vi "Cross Spectrum (Mag-Phase).vi"(0 "time signal X":waveform(dbl), 1 "restart averaging (F)":bool, 2 "window parameter":dbl=nan, 5 "time signal Y":waveform(dbl), 7 "window":T1=1 items=["Rectangle"=0, "Hanning"=1, "Hamming"=2, "Blackman-Harris"=3, "Exact Blackman"=4, "Blackman"=5, "Flat Top"=6, "4 Term B-Harris "=7, "7 Term B-Harris"=8, "Low Sidelobe"=9, "Blackman Nuttall"=11, "Triangle"=30, "Bartlett-Hanning"=31, "Bohman"=32, "Parzen"=33, "Welch"=34, "Kaiser"=60, "Dolph-Chebyshev"=61, "Gaussian"=62], 9 "view":T3, 11 "error in (no error)":errorcluster, 12 "averaging parameters":T2={"averaging mode"=enum."No averaging", "weighting mode"=enum."Exponential", "number of averages"=10} {"number of averages" min=1}) -> (3 "averaging done":bool, 4 "magnitude":cluster{"f0":dbl, "df":dbl, "magnitude":dbl[]} {"magnitude" format="%.2p"; "f0" format="%0.2p"; "df" format="%0.2p"}, 6 "phase":cluster{"f0":dbl, "df":dbl, "phase":dbl[]} {"phase" format="%.2p"; "f0" format="%0.2p"; "df" format="%0.2p"}, 10 "averages completed":dbl format="%.2p", 15 "error out":errorcluster)   [LabVIEW 2020, in "NI_MAPro.lvlib"]
doc: "Computes the averaged cross power spectrum of the input signals. Results are returned as <B>magnitude</B> and <B>phase</B>."
uses:
  NI_MAPro.lvlib
  windowTd.ctl
  NI_AALPro.lvlib
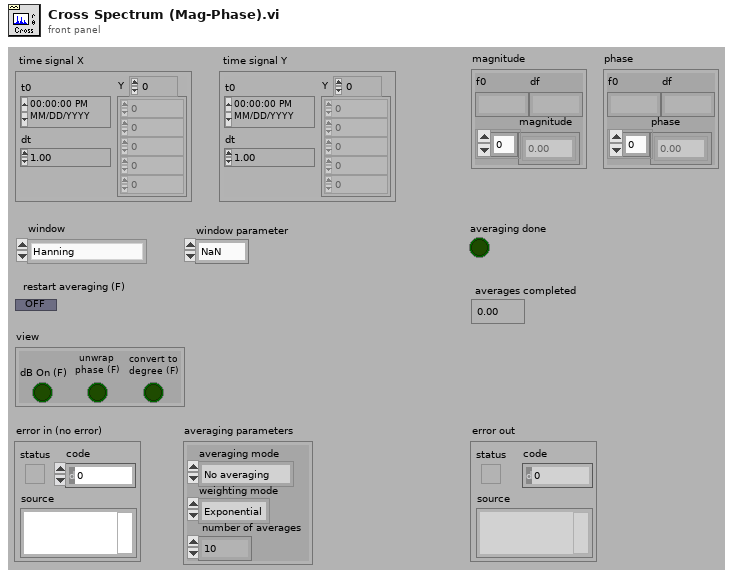
[diagram p1: front panel]
types:
  T1 = typedef "NI_AALPro.lvlib/windowTd.ctl" = u32
  T2 = cluster{"averaging mode":enum16{"No averaging", "Vector averaging", "RMS averaging", "Peak hold"}, "weighting mode":enum16{"Linear", "Exponential"}, "number of averages":u32}
  T3 = cluster{"dB On (F)":bool, "unwrap phase (F)":bool, "convert to degree (F)":bool}
  T4 = enum16{"FFT spectrum", "Power spectrum", "Cross spectrum", "Frequency response"}
  T5 = enum16{"No averaging", "Vector averaging", "RMS averaging", "Peak hold"}
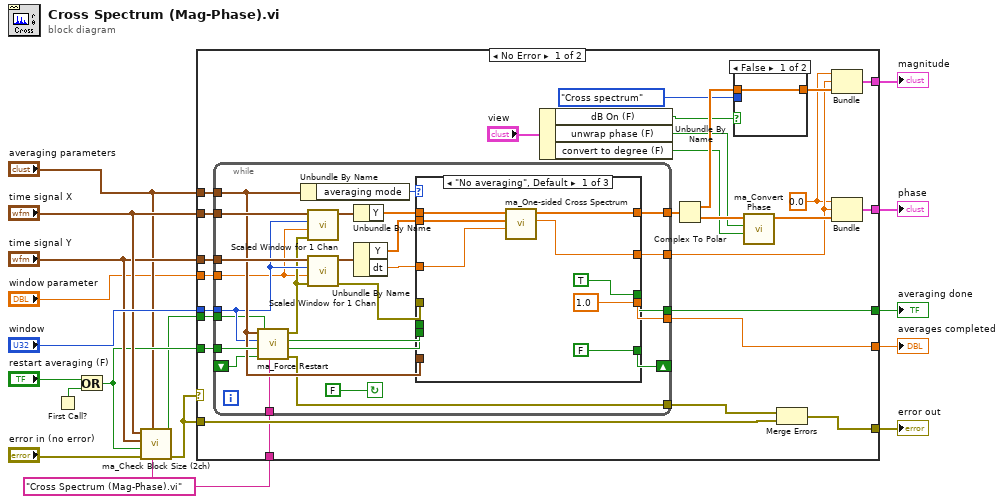
[diagram p0: block diagram]
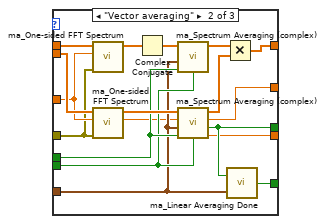
[diagram p2: hidden frame]
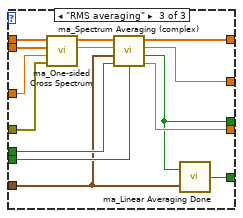
[diagram p3: hidden frame]
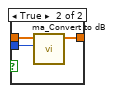
[diagram p4: hidden frame]
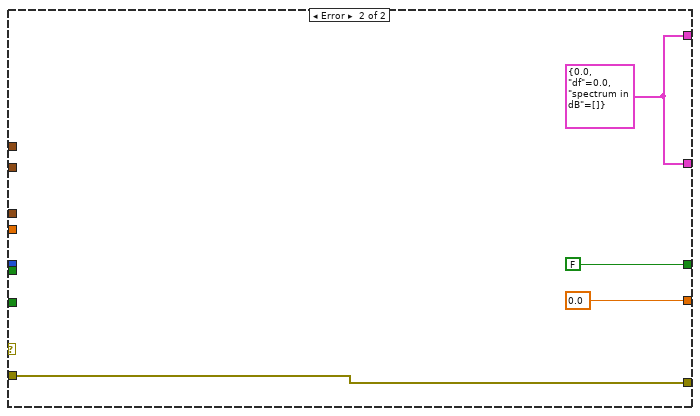
[diagram p5: hidden frame]
diagram:
  w3 = "Cross Spectrum (Mag-Phase).vi" ("caller VI name")
  n1 = First Call?() -> (First Call?: T/F=w7:bool)
  n2 = Or(x="restart averaging (F)", y=w7) -> (x .or. y?=w8:bool)
  n3 = call "ma_Check Block Size (2ch).vi"("caller VI name"=w3, "averaging parameters"="averaging parameters", "error in"="error in (no error)", "restart averaging (F)"=w8, "time signal Y"="time signal Y", "time signal X"="time signal X") -> ("error out"=w9:errorcluster, "force restart averaging"=w2:bool)  [unwired: 4 out]
  n4 = case shown="No Error" w9 {
    tunnel: "averaging parameters" -> [w43 _]
    tunnel: [w41 0.0 ("averages completed")] -> w17
    tunnel: "time signal X" -> [w40 _]
    tunnel: "time signal Y" -> [w39 _]
    tunnel: "window" -> [w38 _]
    tunnel: [w28 w115] -> w5
    tunnel: [w31 FALSE ("averaging done")] -> w15
    tunnel: w8 -> [w30 _]
    tunnel: [w23 w118] -> w14
    tunnel: w9 -> [w21 w118]
    tunnel: [w24 w115] -> w4
    tunnel: w3 -> [w20 _]
    tunnel: w2 -> [w19 _]
    tunnel: "window parameter" -> [w18 _]
    frame No Error {
      w25 = 0.0
      n5 = while {
        tunnel: w20 -> [w47]
        tunnel: [w48] -> w22
        tunnel: w30 -> [w62]
        shift-left: _ -> [w60]
        shift-right: [w64] -> _
        tunnel: [w65] -> w31
        tunnel: w38 -> [w52]
        tunnel: w39 -> [w66]
        tunnel: w40 -> [w67]
        tunnel: [w59] -> w26
        tunnel: [w68] -> w41
        tunnel: [w69] -> w42
        tunnel: w43 -> [w61]
        tunnel: w19 -> [w46]
        tunnel: w18 -> [w45]
        stop <- FALSE continue-if-true
        n6 = call "ma_Force Restart.vi"("caller VI name"=w47, "force restart averaging in"=w46, "linear averaging done"=w60, "restart averaging (F)"=w62, "window"=w52, "averaging parameters"=w61) -> ("error out"=w48:errorcluster, "retrieve last spectrum"=w49:bool, "force restart averaging"=w50:bool, "skip processing"=w51:errorcluster)  [unwired: 2 out]
        n7 = Unbundle By Name(w61) -> ("averaging mode"=w70:T5)
        n8 = call "Scaled Window for 1 Chan.vi"("error in (no error)"=w51, "window parameter"=w45, "window"=w52, "signal in"=w67) -> ("signal out"=w57:waveform(dbl))  [unwired: 5 in, 2 out]
        n9 = call "Scaled Window for 1 Chan.vi"("error in (no error)"=w51, "window parameter"=w45, "window"=w52, "signal in"=w66) -> ("error out"=w63:errorcluster, "signal out"=w53:waveform(dbl))  [unwired: 5 in, 1 out]
        n10 = Unbundle By Name(w57) -> ("Y"=w56:dbl[])
        n11 = Unbundle By Name(w53) -> ("Y"=w55:dbl[], "dt"=w54:dbl)
        n12 = case shown="\"No averaging\", Default" w70 {
          tunnel: w56 -> [w77 w95 w110]
          tunnel: w55 -> [w76 w93 w109]
          tunnel: w54 -> [w75 w92 w108]
          tunnel: [w73 w80 w97] -> w59
          tunnel: [w74 w96 w105] -> w69
          tunnel: w50 -> [_ w88 w106]
          tunnel: w61 -> [_ w83 w101]
          tunnel: [1.0 ("averages completed") w79 w99] -> w68
          tunnel: [TRUE ("averaging done") w82 w98] -> w65
          tunnel: [FALSE ("linear averaging done") w86 w104] -> w64
          tunnel: w63 -> [_ w85 w103]
          tunnel: w49 -> [_ w84 w102]
          frame "No averaging", Default {
            n13 = call "ma_One-sided Cross Spectrum.vi"("dt"=w75, "signal Y (V)"=w76, "signal X (V)"=w77) -> ("df"=w73:dbl, "cross spectrum (V^2 rms)"=w74:cdb[])  [unwired: 1 in, 6 out]
          }
          frame "Vector averaging" {
            n14 = call "ma_One-sided FFT Spectrum.vi"("error in"=w85, "dt"=w92, "signal (V)"=w95) -> ("FFT spectrum (Vrms)"=w94:cdb[])  [unwired: 8 out]
            n15 = call "ma_One-sided FFT Spectrum.vi"("error in"=w85, "dt"=w92, "signal (V)"=w93) -> ("df"=w81:dbl, "FFT spectrum (Vrms)"=w89:cdb[])  [unwired: 7 out]
            n16 = Complex Conjugate(1:w94) -> (0:w91:cdb[])
            n17 = call "ma_Spectrum Averaging (complex).vi"("complex spectrum"=w91, "retrieve last spectrum (F)"=w84, "averaging parameters"=w83, "restart averaging (F)"=w88) -> ("averaged complex spectrum"=w90:cdb[])  [unwired: 1 in, 4 out]
            n18 = call "ma_Spectrum Averaging (complex).vi"("complex spectrum"=w89, "df"=w81, "retrieve last spectrum (F)"=w84, "averaging parameters"=w83, "restart averaging (F)"=w88) -> ("averaged complex spectrum"=w87:cdb[], "df"=w80:dbl, "averaging done"=w82:bool, "averages completed"=w79:dbl)  [unwired: 1 out]
            n19 = Multiply(x=w90, y=w87) -> (x*y=w96:cdb[])
            n20 = call "ma_Linear Averaging Done.vi"("averaging parameters"=w83, "averaging done"=w82) -> ("linear averaging done"=w86:bool)
          }
          frame "RMS averaging" {
            n21 = call "ma_One-sided Cross Spectrum.vi"("error in"=w103, "dt"=w108, "signal Y (V)"=w109, "signal X (V)"=w110) -> ("df"=w100:dbl, "cross spectrum (V^2 rms)"=w107:cdb[])  [unwired: 6 out]
            n22 = call "ma_Spectrum Averaging (complex).vi"("complex spectrum"=w107, "df"=w100, "retrieve last spectrum (F)"=w102, "averaging parameters"=w101, "restart averaging (F)"=w106) -> ("averaged complex spectrum"=w105:cdb[], "df"=w97:dbl, "averaging done"=w98:bool, "averages completed"=w99:dbl)  [unwired: 1 out]
            n23 = call "ma_Linear Averaging Done.vi"("averaging parameters"=w101, "averaging done"=w98) -> ("linear averaging done"=w104:bool)
          }
        }
      }
      n24 = Unbundle By Name("view") -> ("dB On (F)"=w36:bool, "unwrap phase (F)"=w33:bool, "convert to degree (F)"=w32:bool)
      n25 = Complex To Polar(r * e^(i*theta)=w42) -> (r=w37:dbl[], theta=w34:dbl[])
      n26 = case shown="False" w36 {
        tunnel: [w111 w113] -> w29
        tunnel: w37 -> [w111 w114]
        tunnel: T4."Cross spectrum" ("spectrum type") -> [_ w112]
        frame False {
        }
        frame True {
          n27 = call "ma_Convert to dB.vi"("spectrum type"=w112, "spectrum"=w114) -> ("spectrum in dB"=w113:dbl[])  [unwired: 9 out]
        }
      }
      n28 = call "ma_Convert Phase.vi"("convert to degree (F)"=w32, "unwrap phase (F)"=w33, "phase (radian)"=w34) -> ("scaled phase"=w27:dbl[])  [unwired: 3 in, 5 out]
      n29 = Merge Errors(w22, w21) -> (w23:errorcluster)
      n30 = Bundle(w25, "df"=w26, "spectrum in dB"=w29) -> (w28:cluster{dbl, "df":dbl, "spectrum in dB":dbl[]})  [unwired: 1 out]
      n31 = Bundle(w25, "df"=w26, "scaled phase"=w27) -> (w24:cluster{dbl, "df":dbl, "scaled phase":dbl[]})  [unwired: 1 out]
    }
    frame Error {
      w115 = cluster{dbl, "df":dbl, "spectrum in dB":dbl[]} {0.0, "df"=0.0, "spectrum in dB"=[]}
    }
  }
  "averages completed" <- w17
  "error out" <- w14
  "averaging done" <- w15
  "magnitude" <- w5
  "phase" <- w4
